vi "OldControlFiles.vi"() -> ()   [LabVIEW 2013]
uses:
  <vilib>/DAQmx/write.llb/DAQmx Write (Analog 1D DBL 1Chan NSamp).vi
  <vilib>/Utility/file.llb/Read From Spreadsheet File (DBL).vi
  <vilib>/DAQmx/create/channels.llb/DAQmx Create Channel (AO-Voltage-Basic).vi
  <vilib>/DAQmx/configure/timing.llb/DAQmx Timing (Sample Clock).vi
  <vilib>/DAQmx/miscellaneous.llb/DAQmx Fill In Error Info.vi
  <resource>/objmgr/daqmx.rc
panel:
  out "Control Graph":T1(graph)
  out "Actual Clock Rate":dbl
  out "Total Samples":i32
  out "Total Time [minutes]":dbl format="%.2f"
  in  "Update Rate [Hz]":dbl=10.0
  # "Instructions:\n\n1) Set the update rate in the VI\n2) Click the run arrow\n3) Select the desired control file\n4) Prepare your experiment and lock the piston\n5) Start the file and a stopwatch\n6) Plug in the control signal and zero the pointer\n7) Unlock the piston\n\nVersion 1.0.1\nJ.R. Leeman\nkd5wxb@gmail.com"
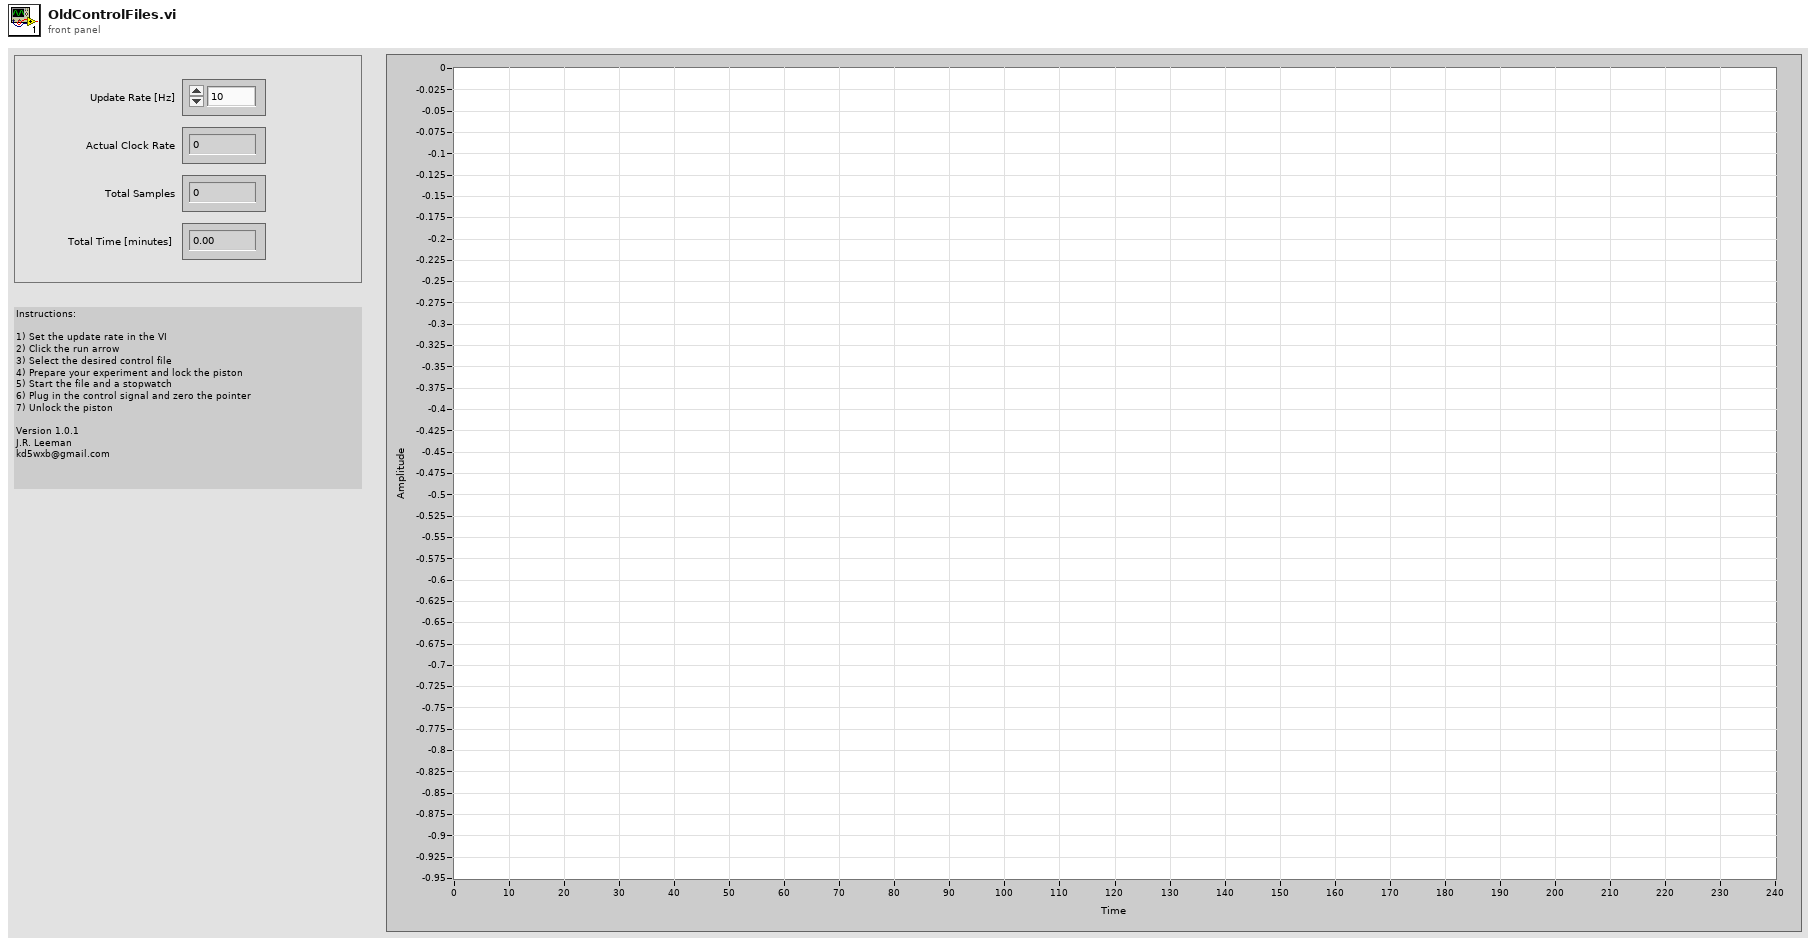
[diagram p1: front panel]
types:
  T1 = cluster{"minimum value":dbl, dbl, "all rows":dbl[]}
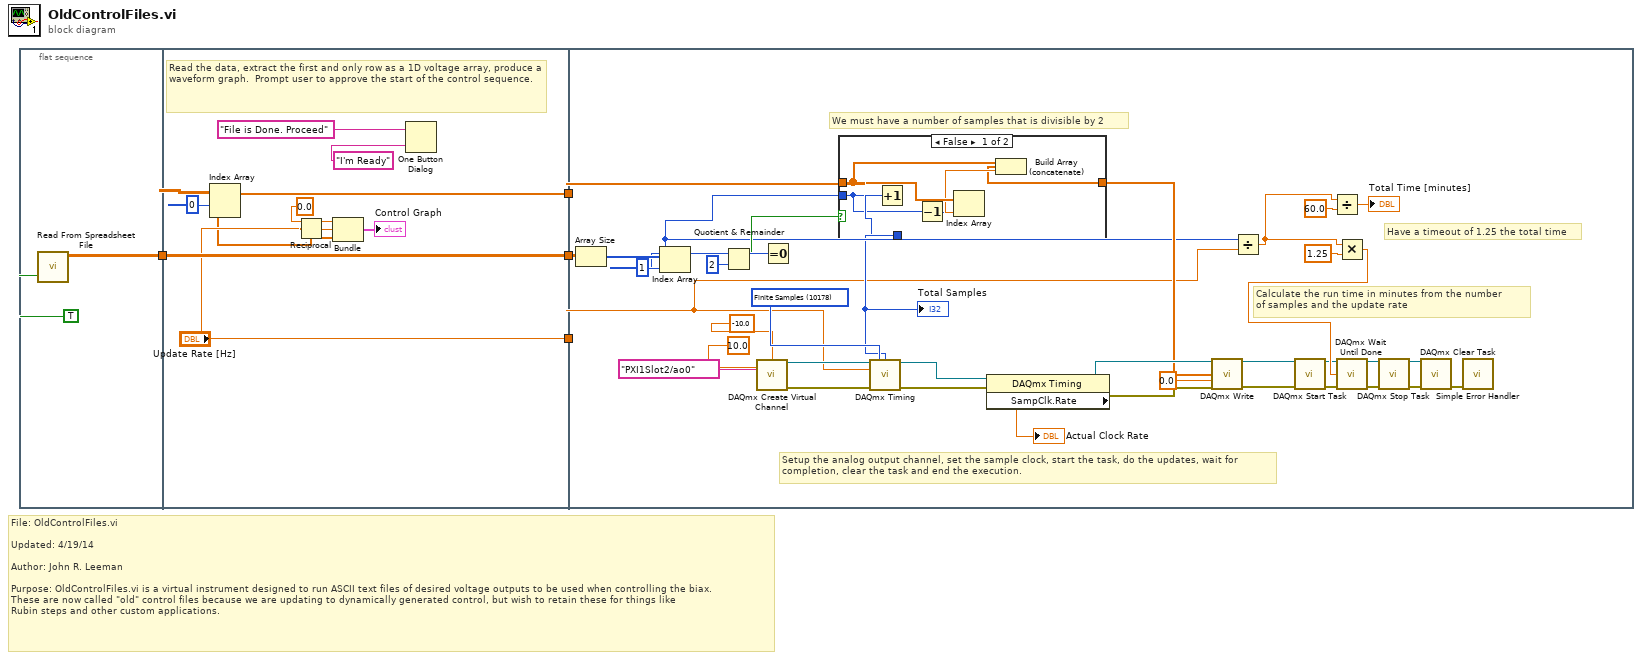
[diagram p0: block diagram]
diagram:
  # "File: OldControlFiles.vi\n\nUpdated: 4/19/14\n\nAuthor: John R. Leeman\n\nPurpose: OldControlFiles.vi is a virtual instrument designed to run ASCII text files of desired voltage outputs to be used when controlling the biax.\nThese are now called \"old\" control files because we are updating to dynamically generated control, but wish to retain these for things like\nRubin steps and other custom applications."
  n1 = flat-sequence {
    tunnel: [w5] -> w4
    tunnel: w4 -> [w12]
    tunnel: [w12] -> w3
    tunnel: ["Update Rate [Hz]"] -> w2
    tunnel: [w7] -> w1
    tunnel: w3 -> [w35]
    tunnel: w2 -> [w17]
    tunnel: w1 -> [w16]
    frame #0 {
      n2 = call-poly <vilib>:"Read From Spreadsheet File.vi"("transpose (no:F)"=TRUE) -> ("all rows"=w5:dbl[][])  [unwired: 6 in, 4 out]
    }
    frame #1 {
      # "Read the data, extract the first and only row as a 1D voltage array, produce a waveform graph.  Prompt user to approve the start of the control sequence."
      n3 = Index Array(array=w12, index (row)=0) -> (element=w7:dbl[])  [unwired: 1 in]
      n4 = Reciprocal(x="Update Rate [Hz]") -> (1/x=w11:dbl)
      n5 = Bundle("minimum value"=0.0, w11, "all rows"=w7) -> (→"Control Graph":T1)  [unwired: 1 in]
      n6 = One Button Dialog(message="File is Done. Proceed", button name ("OK")="I'm Ready") -> ()  [unwired: 1 out]
    }
    frame #2 {
      w48 = 10178 items=["Finite Samples"=10178, "Continuous Samples"=10123, "Hardware Timed Single Point"=12522] ("sample mode")
      # "Have a timeout of 1.25 the total time"
      # "We must have a number of samples that is divisible by 2"
      # "Setup the analog output channel, set the sample clock, start the task, do the updates, wait for \ncompletion, clear the task and end the execution."
      # "Calculate the run time in minutes from the number \nof samples and the update rate"
      n7 = Array Size(array=w35) -> (size(s)=w47:i32[])
      n8 = Index Array(array=w47, index=1) -> (element=w19:i32)
      n9 = Quotient & Remainder(x=w19, y=2) -> (x-y*floor(x/y)=w22:i32)  [unwired: 1 out]
      n10 = call-poly <vilib>:"DAQmx Create Virtual Channel.vi"("maximum value"=10.0, "minimum value"=-10.0, "physical channels"=tag "PXI1Slot2/ao0") -> ("task out"=w52:refnum<k21>, "error out"=w51:errorcluster)  [unwired: 11 in]
      n11 = Equal To 0?(x=w22) -> (x = 0?=w21:bool)
      n12 = case shown="False" w21 {
        tunnel: w16 -> [w56 w60]
        tunnel: [w54 w60] -> w20
        tunnel: [w58 w59] -> w18
        tunnel: w19 -> [w57 w59]
        frame False {
          n13 = Increment(x=w57) -> (x+1=w58:i32)
          n14 = Decrement(x=w57) -> (x-1=w53:i32)
          n15 = Index Array(array=w56, index=w53) -> (element=w55:dbl)
          n16 = Build Array (concatenate)(w56, w55) -> (w54:dbl[])
        }
        frame True {
        }
      }
      "Total Samples" <- w18
      n17 = call-poly <vilib>:"DAQmx Timing.vi"("task/channels in"=w52, "sample mode"=w48, "samples per channel"=w18, "rate"=w17, "error in"=w51) -> ("task out"=w34:refnum<k21>, "error out"=w31:errorcluster)  [unwired: 9 in]
      n18 = property class="DAQmx Timing"(reference=w34, error in=w31) -> (reference out=w29:refnum<k21>, error out=w28:errorcluster, "SampClk.Rate"=→"Actual Clock Rate":dbl)
      n19 = call-poly <vilib>:"DAQmx Write.vi"("task/channels in"=w29, "data"=w20, "timeout"=0.0, "error in"=w28) -> ("task out"=w27:refnum<k21>, "error out"=w24:errorcluster)  [unwired: 9 in, 1 out]
      n20 = Divide(x=w19, y=w17) -> (x/y=w43:dbl)
      n21 = call <vilib>:"DAQmx Start Task.vi"("task/channels in"=w27, "error in"=w24) -> ("task out"=w26:refnum<k21>, "error out"=w25:errorcluster)  [unwired: 12 in]
      n22 = Divide(x=w43, y=60.0) -> (x/y=→"Total Time [minutes]":dbl)
      n23 = Multiply(x=w43, y=1.25) -> (x*y=w42:dbl)
      n24 = call <vilib>:"DAQmx Wait Until Done.vi"("task/channels in"=w26, "timeout (sec)"=w42, "error in"=w25) -> ("task out"=w33:refnum<k21>, "error out"=w38:errorcluster)  [unwired: 11 in]
      n25 = call <vilib>:"DAQmx Stop Task.vi"("task/channels in"=w33, "error in"=w38) -> ("task out"=w32:refnum<k21>, "error out"=w39:errorcluster)  [unwired: 12 in]
      n26 = call <vilib>:"DAQmx Clear Task.vi"("task in"=w32, "error in"=w39) -> ("error out"=w50:errorcluster)  [unwired: 13 in]
      n27 = call <vilib>:"Simple Error Handler.vi"("error in (no error)"=w50) -> ()  [unwired: 4 in, 5 out]
    }
  }
